vi "plot Timeout Helper.vi"(5 "new timeout?":bool, 7 "new timeout mS":i32, 11 "Timeout":i32) -> (3 "Timeout":i32)   [LabVIEW 2021, in "RocketPlot.lvlib"]
uses:
  RocketPlot.lvlib
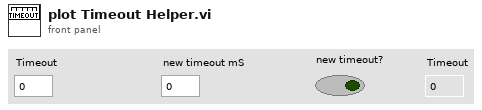
[diagram p1: front panel]
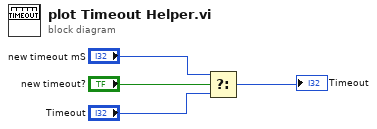
[diagram p0: block diagram]
diagram:
  n1 = Select(t="new timeout mS", s="new timeout?", f="Timeout") -> (s? t:f=→"Timeout":i32)
